vi "get data definition.vi"(10 "channel classification":T1, 11 "fixed channel runtime in":refnum<class "user control module.lvclass">) -> (1 "valid?":bool, 2 "index cluster":variant, 3 "fixed channel runtime out":refnum<class "user control module.lvclass">)   [LabVIEW 2013, in "user control module.lvclass"]
uses:
  user control module.lvclass
  input user data.ctl
  output user data.ctl
  parameter user data.ctl
  result user data.ctl
  <vilib>/NI/Tag Bus Module Framework/channel/channel classification.ctl
  <vilib>/NI/Tag Bus Module Framework/channel/TBM channel.lvclass
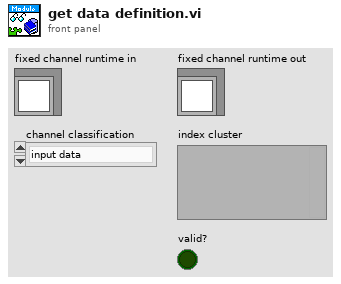
[diagram p1: front panel]
types:
  T1 = typedef "TBM channel.lvclass/channel classification.ctl" = enum16{"input data", "output data", "processing parameter", "processing result"}
  T2 = typedef "user control module.lvclass/input user data.ctl" = cluster{"fmwk_placeholder":sgl}
  T3 = typedef "user control module.lvclass/output user data.ctl" = cluster{"fmwk_placeholder":sgl}
  T4 = typedef "user control module.lvclass/parameter user data.ctl" = cluster{"fmwk_placeholder":sgl}
  T5 = typedef "user control module.lvclass/result user data.ctl" = cluster{"fmwk_placeholder":sgl}
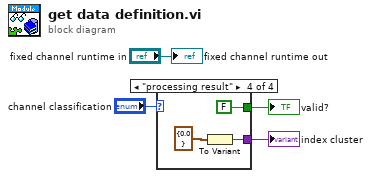
[diagram p0: block diagram]
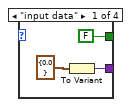
[diagram p2: hidden frame]
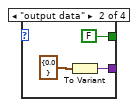
[diagram p3: hidden frame]
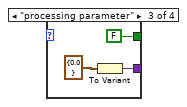
[diagram p4: hidden frame]
diagram:
  n1 = case shown="\"processing result\"" "channel classification" {
    tunnel: [w6 w10 w13 w16] -> w2
    tunnel: [FALSE FALSE FALSE FALSE] -> w1
    frame "input data" {
      n2 = To Variant(anything=T2 {"fmwk_placeholder"=0.0} ("Inputs from system")) -> (Variant=w6:variant)
    }
    frame "output data" {
      n3 = To Variant(anything=T3 {"fmwk_placeholder"=0.0} ("Outputs to system")) -> (Variant=w10:variant)
    }
    frame "processing parameter" {
      n4 = To Variant(anything=T4 {"fmwk_placeholder"=0.0} ("Parameters to process")) -> (Variant=w13:variant)
    }
    frame "processing result" {
      n5 = To Variant(anything=T5 {"fmwk_placeholder"=0.0} ("Results from processing")) -> (Variant=w16:variant)
    }
  }
  "index cluster" <- w2
  "valid?" <- w1
  "fixed channel runtime out" <- "fixed channel runtime in"
